vi "write_data_to_CSV.vi"(0 "file path (dialog if empty)":path, 7 "Show mass domain?":bool, 11 "error in (no error)":errorcluster, 12 "Time data":dbl[](array[numeric]), 13 "Intensity data":dbl[](array[numeric]), 14 "Mass data":dbl[](array[numeric])) -> (15 "error out":errorcluster)   [LabVIEW 2023]
uses:
  <vilib>/Utility/file.llb/Write Delimited Spreadsheet (DBL).vi
  <vilib>/Utility/file.llb/Write Delimited Spreadsheet (string).vi
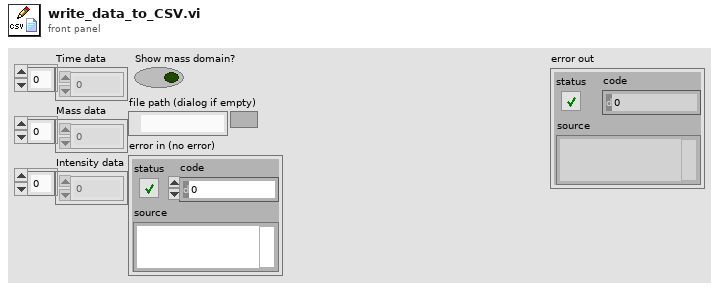
[diagram p1: front panel]
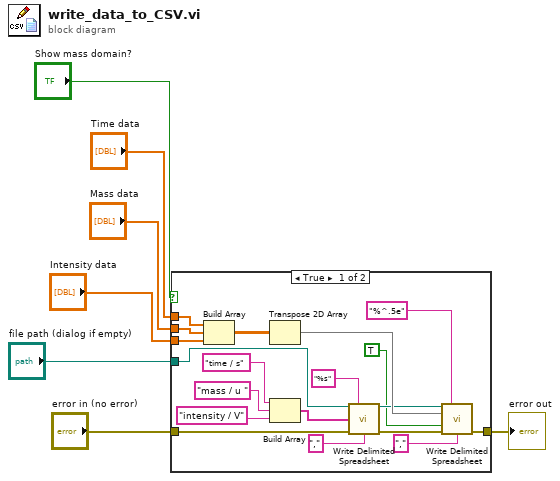
[diagram p0: block diagram]
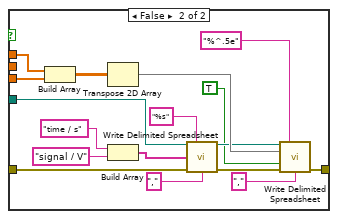
[diagram p2: hidden frame]
diagram:
  n1 = case shown="True" "Show mass domain?" {
    tunnel: "file path (dialog if empty)" -> [w24 w41]
    tunnel: "Time data" -> [w13 w32]
    tunnel: "Mass data" -> [w12 _]
    tunnel: "Intensity data" -> [w11 w30]
    tunnel: "error in (no error)" -> [w9 w28]
    tunnel: [w8 w27] -> w1
    frame True {
      n2 = Build Array(w13, w12, w11) -> (w10:dbl[][])
      n3 = Transpose 2D Array(2D array=w10) -> (transposed array=w25:dbl[][])
      n4 = Build Array("time / s", "mass / u ", "intensity / V") -> (w17:string[])
      n5 = call-poly <vilib>:"Write Delimited Spreadsheet.vi"("file path (dialog if empty)"=w24, "format (%s)"="%s", "1D data"=w17, "error in (no error)"=w9, "delimiter (\\t)"="," ("delimiter (\\t)")) -> ("new file path (Not A Path if cancelled)"=w23:path, "error out"=w16:errorcluster)  [unwired: 9 in]
      n6 = call-poly <vilib>:"Write Delimited Spreadsheet.vi"("file path (dialog if empty)"=w23, "format (%.3f)"="%^.5e", "2D data"=w25, "append to file? (new file:F)"=TRUE, "error in (no error)"=w16, "delimiter (\\t)"="," ("delimiter (\\t)")) -> ("error out"=w8:errorcluster)  [unwired: 8 in, 1 out]
    }
    frame False {
      n7 = Build Array(w32, w30) -> (w31:dbl[][])
      n8 = Transpose 2D Array(2D array=w31) -> (transposed array=w42:dbl[][])
      n9 = Build Array("time / s", "signal / V") -> (w36:string[])
      n10 = call-poly <vilib>:"Write Delimited Spreadsheet.vi"("file path (dialog if empty)"=w41, "format (%s)"="%s", "1D data"=w36, "error in (no error)"=w28, "delimiter (\\t)"="," ("delimiter (\\t)")) -> ("new file path (Not A Path if cancelled)"=w40:path, "error out"=w35:errorcluster)  [unwired: 9 in]
      n11 = call-poly <vilib>:"Write Delimited Spreadsheet.vi"("file path (dialog if empty)"=w40, "format (%.3f)"="%^.5e", "2D data"=w42, "append to file? (new file:F)"=TRUE, "error in (no error)"=w35, "delimiter (\\t)"="," ("delimiter (\\t)")) -> ("error out"=w27:errorcluster)  [unwired: 8 in, 1 out]
    }
  }
  "error out" <- w1
